vi "Excel Select Worksheet.vi"(11 "Excel._Application":refnum<k7>) -> (0 "Canceled":bool=TRUE, 1 "Excel._Worksheet TRANS":refnum<k7>, 2 "Excel._Worksheet SINE":refnum<k7>, 3 "Excel._Application":refnum<k7>)   [LabVIEW 2016]
panel:
  in  "Excel._Worksheet TRANS":refnum<k7>
  in  "Text":bool
  in  "Excel._Worksheet SINE":refnum<k7>
  in  "Cancel":bool
  in  "OK Button":bool
  # "Please sellect now the worksheet that you \nwould like to use for saving the \n                             data.\n\nWhen you are done press OK"
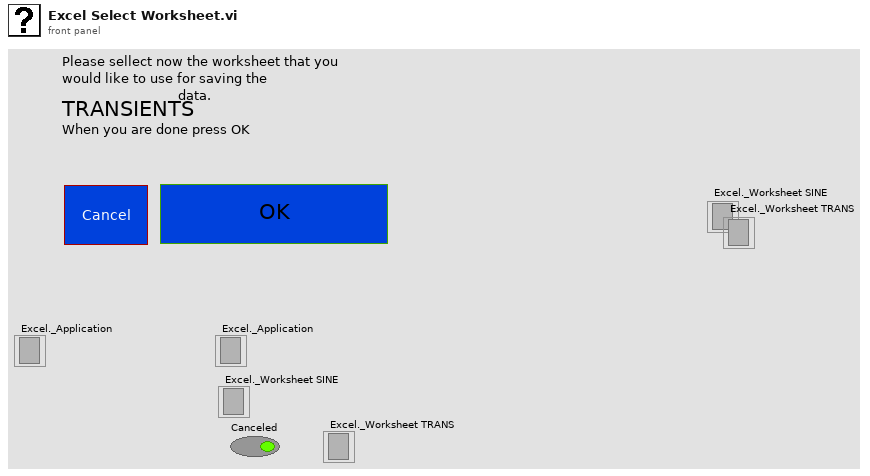
[diagram p1: front panel]
types:
  T1 = cluster{"Excel._Application":refnum<k7>, "Excel._Worksheet SINE":refnum<k7>, "Excel._Worksheet TRANS":refnum<k7>}
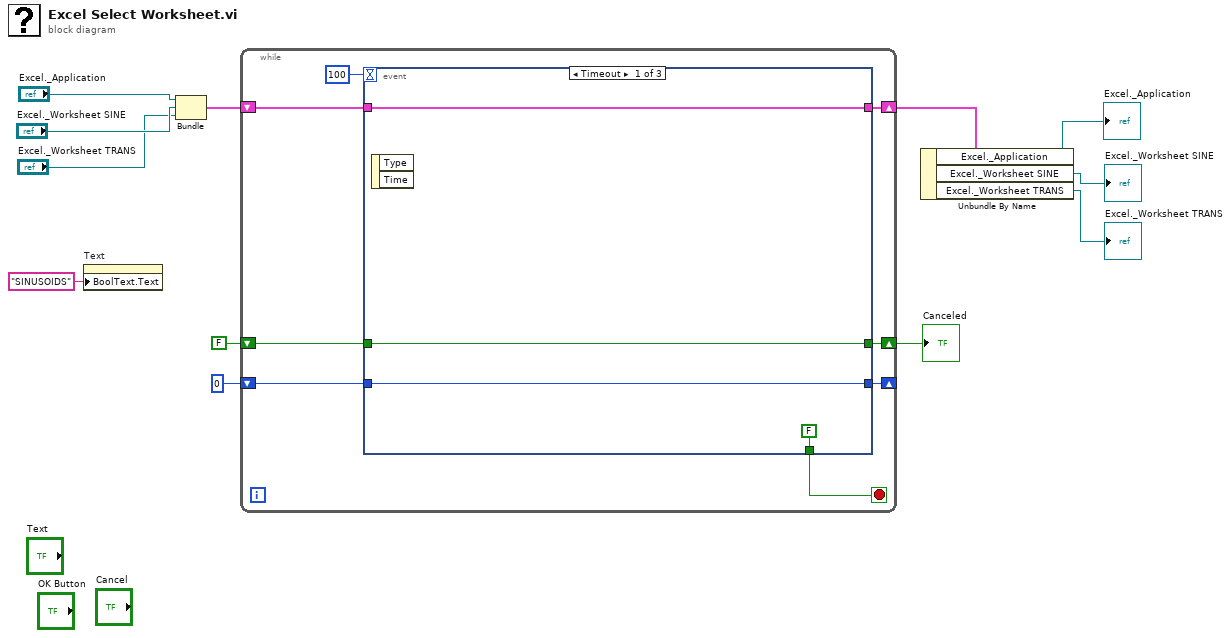
[diagram p0: block diagram]
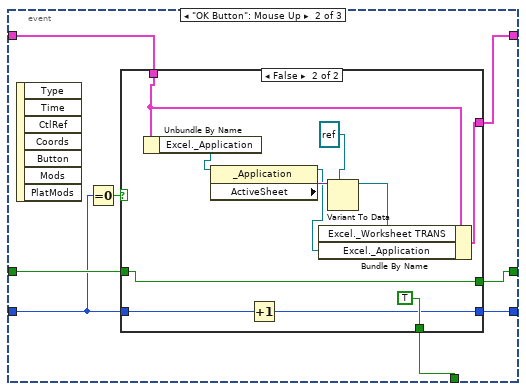
[diagram p2: hidden frame]
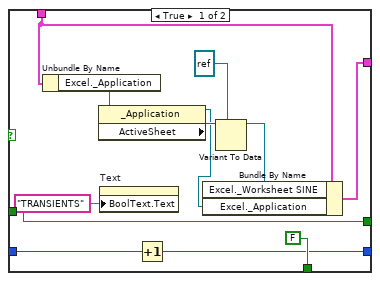
[diagram p3: hidden frame]
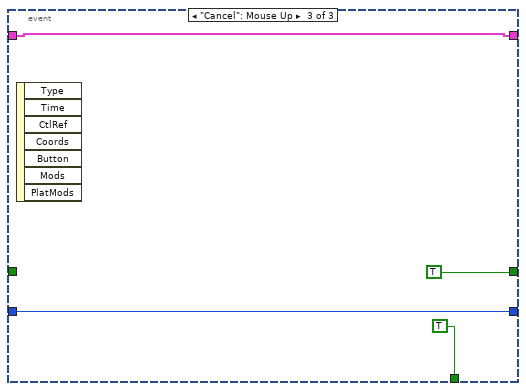
[diagram p4: hidden frame]
diagram:
  n1 = property on="Text" class="Bool"("BoolText.Text"="SINUSOIDS" ("Boolean Text.Text")) -> ()  [unwired: 2 in, 2 out]
  n2 = Bundle("Excel._Application"="Excel._Application", "Excel._Worksheet SINE"="Excel._Worksheet SINE", "Excel._Worksheet TRANS"="Excel._Worksheet TRANS") -> (w6:T1)  [unwired: 1 in]
  n3 = while {
    shift-right: [w15] -> w10
    shift-left: FALSE -> [w18]
    shift-right: [w16] -> _
    shift-left: 0 -> [w17]
    shift-right: [w13] -> w5
    shift-left: w6 -> [w14]
    stop <- w19 stop-if-true
    n4 = event shown="[0] Timeout" {
      selector: _ -> [_ _ _]
      dyn-events: _ -> [_ _ _]
      timeout: 100 -> [_ _ _]
      tunnel: [FALSE w32 TRUE] -> w19
      tunnel: w18 -> [w22 w31 _]
      tunnel: w17 -> [w23 w29 w58]
      tunnel: [w23 w28 w58] -> w16
      tunnel: [w22 w25 TRUE] -> w15
      tunnel: w14 -> [w21 w27 w56]
      tunnel: [w21 w26 w56] -> w13
      event Timeout {
        n5 = event-data() -> ()  [unwired: 1 in, 2 out]
      }
      event "OK Button": Mouse Up {
        n6 = event-data() -> ()  [unwired: 1 in, 7 out]
        n7 = Equal To 0?(x=w29) -> (x = 0?=w30:bool)
        n8 = case shown="False" w30 {
          tunnel: [FALSE TRUE] -> w32
          tunnel: w31 -> [w35 w46]
          tunnel: w29 -> [w42 w53]
          tunnel: [w41 w52] -> w28
          tunnel: w27 -> [w38 w50]
          tunnel: [w39 w49] -> w26
          tunnel: [w35 w46] -> w25
          frame True {
            n9 = Unbundle By Name(w38) -> ("Excel._Application"=w40:refnum<k7>)
            n10 = property class="_Application"(reference=w40) -> (reference out=w36:refnum<k7>, "ActiveSheet"=w44:variant)  [unwired: 1 in, 1 out]
            n11 = property on="Text" class="Bool"("BoolText.Text"="TRANSIENTS" ("Boolean Text.Text")) -> ()  [unwired: 2 in, 2 out]
            n12 = Increment(x=w42) -> (x+1=w41:i32)
            n13 = Variant To Data(type=refnum<k7> refnum ("Excel._Worksheet SINE"), Variant=w44) -> (data=w37:refnum<k7>)  [unwired: 1 in, 1 out]
            n14 = Bundle By Name(cluster=w38, "Excel._Worksheet SINE"=w37, "Excel._Application"=w36) -> (w39:T1)
          }
          frame False {
            n15 = Unbundle By Name(w50) -> ("Excel._Application"=w51:refnum<k7>)
            n16 = property class="_Application"(reference=w51) -> (reference out=w47:refnum<k7>, "ActiveSheet"=w55:variant)  [unwired: 1 in, 1 out]
            n17 = Increment(x=w53) -> (x+1=w52:i32)
            n18 = Variant To Data(type=refnum<k7> refnum ("Excel._Worksheet SINE"), Variant=w55) -> (data=w48:refnum<k7>)  [unwired: 1 in, 1 out]
            n19 = Bundle By Name(cluster=w50, "Excel._Worksheet TRANS"=w48, "Excel._Application"=w47) -> (w49:T1)
          }
        }
      }
      event "Cancel": Mouse Up {
        n20 = event-data() -> ()  [unwired: 1 in, 7 out]
      }
    }
  }
  "Canceled" <- w10
  n21 = Unbundle By Name(w5) -> ("Excel._Application"=→"Excel._Application":refnum<k7>, "Excel._Worksheet SINE"=→"Excel._Worksheet SINE":refnum<k7>, "Excel._Worksheet TRANS"=→"Excel._Worksheet TRANS":refnum<k7>)
